vi "Check Calibration Point.vi"(0 "Steady State Duration":i32, 1 "Channel":i32, 5 "Maximum Settling Timeout":i32=8, 7 "Pass Flag?":bool, 9 "Reset?":bool, 11 "error in (no error)":errorcluster, 12 "Number of Channels":i32) -> (4 "Record?":bool, 6 "Test Status":T1, 15 "error out":errorcluster)   [LabVIEW 2026, in "Processing_Engine.lvlib"]
uses:
  Processing_Engine.lvlib
  Test Status.ctl
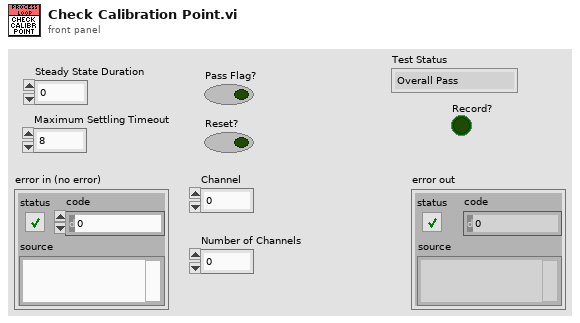
[diagram p1: front panel]
types:
  T1 = typedef "Test Status.ctl" = enum16{"Overall Pass", "Overall Fail", "Test Running"}
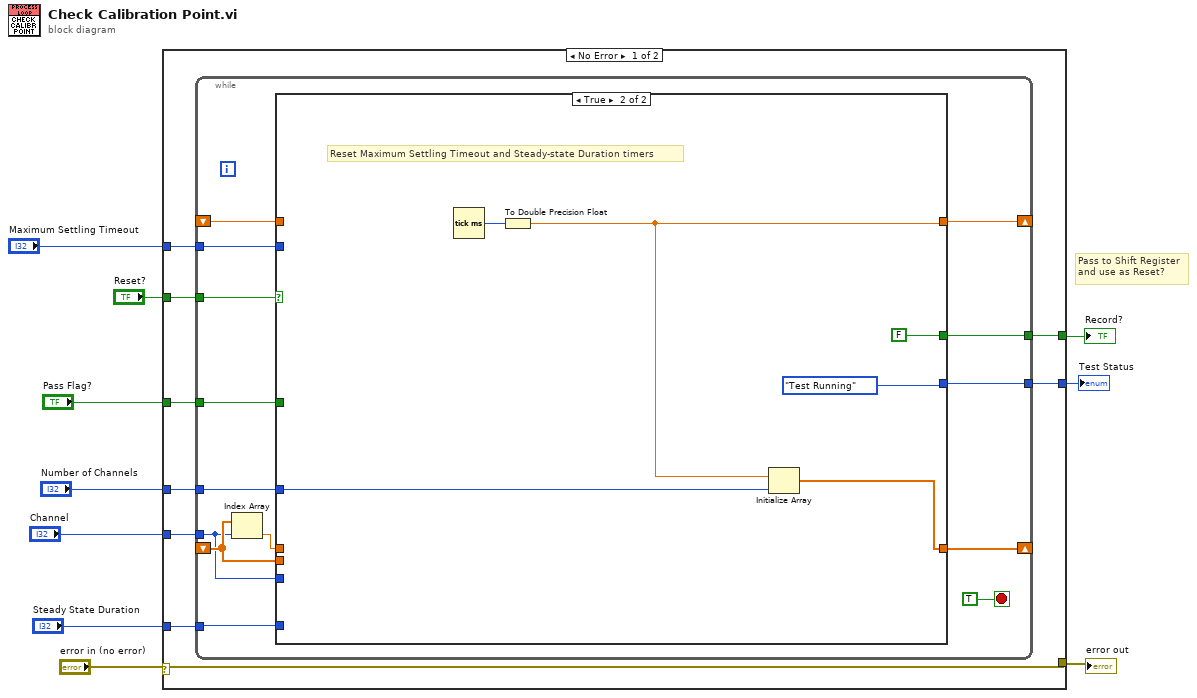
[diagram p0: block diagram]
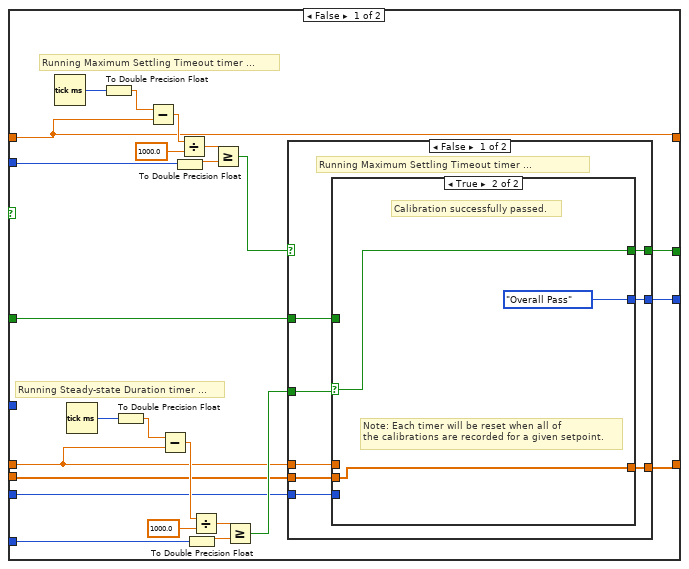
[diagram p2: hidden frame]
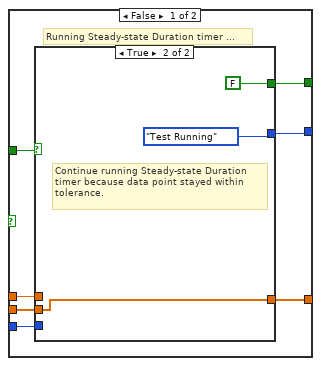
[diagram p3: hidden frame]
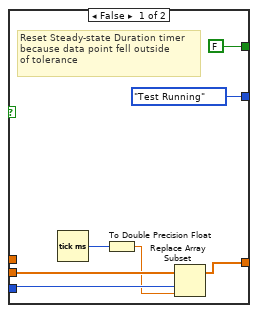
[diagram p4: hidden frame]
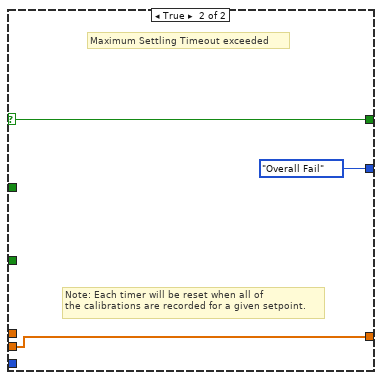
[diagram p5: hidden frame]
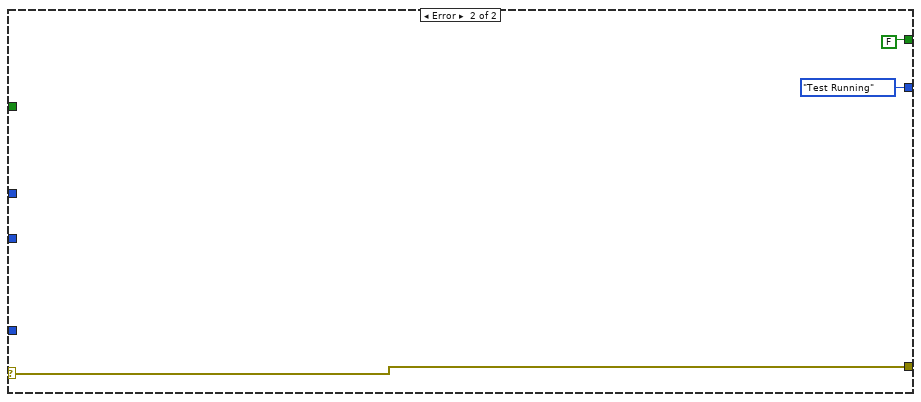
[diagram p6: hidden frame]
diagram:
  # "Pass to Shift Register\nand use as Reset?"
  n1 = case shown="No Error" "error in (no error)" {
    selector: "error in (no error)" -> [w16 w97]
    tunnel: "Maximum Settling Timeout" -> [w19 _]
    tunnel: "Pass Flag?" -> [w18 _]
    tunnel: [w17 FALSE] -> w9
    tunnel: [w16 w97] -> w7
    tunnel: "Reset?" -> [w15 _]
    tunnel: "Steady State Duration" -> [w14 _]
    tunnel: "Channel" -> [w12 _]
    tunnel: "Number of Channels" -> [w13 _]
    tunnel: [w11 Test_Status."Test Running"] -> w1
    frame No Error {
      n2 = while {
        tunnel: w19 -> [w30]
        tunnel: w18 -> [w27]
        shift-right: [w32] -> _
        shift-left: _ -> [w31]
        tunnel: [w29] -> w17
        tunnel: w15 -> [w28]
        shift-right: [w26] -> _
        shift-left: _ -> [w22]
        tunnel: w14 -> [w25]
        tunnel: w13 -> [w24]
        tunnel: w12 -> [w21]
        tunnel: [w20] -> w11
        stop <- TRUE stop-if-true
        n3 = Index Array(array=w22, index=w21) -> (element=w23:dbl)
        n4 = case shown="True" w28 {
          tunnel: [w50 w91] -> w32
          tunnel: w31 -> [w50 _]
          tunnel: w30 -> [w55 _]
          tunnel: [w49 FALSE] -> w29
          tunnel: w27 -> [w47 _]
          tunnel: [w38 w90] -> w26
          tunnel: w25 -> [w40 _]
          tunnel: w23 -> [w37 _]
          tunnel: w24 -> [_ w92]
          tunnel: w22 -> [w36 _]
          tunnel: w21 -> [w35 _]
          tunnel: [w34 Test_Status."Test Running"] -> w20
          frame False {
            # "Running Steady-state Duration timer ..."
            # "Running Maximum Settling Timeout timer ..."
            n5 = Tick Count (ms)() -> (millisecond timer value=w52:u32)
            n6 = Tick Count (ms)() -> (millisecond timer value=w42:u32)
            n7 = To Double Precision Float(number=w52) -> (double precision float=w51:dbl)
            n8 = To Double Precision Float(number=w42) -> (double precision float=w41:dbl)
            n9 = Subtract(x=w51, y=w50) -> (x-y=w53:dbl)
            n10 = Subtract(x=w41, y=w37) -> (x-y=w43:dbl)
            n11 = To Double Precision Float(number=w55) -> (double precision float=w54:dbl)
            n12 = Divide(x=w53, y=1000.0) -> (x/y=w56:dbl)
            n13 = To Double Precision Float(number=w40) -> (double precision float=w44:dbl)
            n14 = Divide(x=w43, y=1000.0) -> (x/y=w45:dbl)
            n15 = Greater Or Equal?(x=w56, y=w54) -> (x >= y?=w48:bool)
            n16 = Greater Or Equal?(x=w45, y=w44) -> (x >= y?=w39:bool)
            n17 = case shown="False" w48 {
              selector: w48 -> [_ w87]
              tunnel: [w64 w87] -> w49
              tunnel: w47 -> [w63 _]
              tunnel: w39 -> [w65 _]
              tunnel: [w62 w88] -> w38
              tunnel: w37 -> [w61 _]
              tunnel: w36 -> [w60 w88]
              tunnel: w35 -> [w59 _]
              tunnel: [w58 Test_Status."Overall Fail"] -> w34
              frame False {
                # "Running Maximum Settling Timeout timer ..."
                n18 = case shown="True" w65 {
                  selector: w65 -> [_ w84]
                  tunnel: [w69 w84] -> w64
                  tunnel: w63 -> [w72 _]
                  tunnel: [w71 w85] -> w62
                  tunnel: w61 -> [w70 _]
                  tunnel: w60 -> [w68 w85]
                  tunnel: w59 -> [w67 _]
                  tunnel: [w66 Test_Status."Overall Pass"] -> w58
                  frame False {
                    # "Running Steady-state Duration timer ..."
                    n19 = case shown="True" w72 {
                      tunnel: [w74 w81] -> w71
                      tunnel: w70 -> [_ _]
                      tunnel: [FALSE FALSE] -> w69
                      tunnel: w68 -> [w77 w81]
                      tunnel: w67 -> [w76 _]
                      tunnel: [Test_Status."Test Running" Test_Status."Test Running"] -> w66
                      frame False {
                        # "Reset Steady-state Duration timer \nbecause data point fell outside \nof tolerance"
                        n20 = Tick Count (ms)() -> (millisecond timer value=w79:u32)
                        n21 = To Double Precision Float(number=w79) -> (double precision float=w75:dbl)
                        n22 = Replace Array Subset(array=w77, new element=w75, index=w76) -> (w74:dbl[])
                      }
                      frame True {
                        # "Continue running Steady-state Duration\ntimer because data point stayed within\ntolerance."
                      }
                    }
                  }
                  frame True {
                    # "Note: Each timer will be reset when all of \nthe calibrations are recorded for a given setpoint."
                    # "Calibration successfully passed."
                  }
                }
              }
              frame True {
                # "Note: Each timer will be reset when all of \nthe calibrations are recorded for a given setpoint."
                # "Maximum Settling Timeout exceeded"
              }
            }
          }
          frame True {
            # "Reset Maximum Settling Timeout and Steady-state Duration timers"
            n23 = Tick Count (ms)() -> (millisecond timer value=w94:u32)
            n24 = To Double Precision Float(number=w94) -> (double precision float=w91:dbl)
            n25 = Initialize Array(w91, w92) -> (w90:dbl[])
          }
        }
      }
    }
    frame Error {
    }
  }
  "Record?" <- w9
  "error out" <- w7
  "Test Status" <- w1
